vi "Go.vi"(6 "assembly type":string, 8 "First?":bool, 9 "Timing Data":T1(array[cluster]), 10 "Control In":T2={"I-O.lvclass"=refnum, "Gantry"=refnum, "Dispenser"="COM1"}, 11 "Dispense in":refnum<class "Dispense.lvclass">) -> (2 "Control Out":T2={"I-O.lvclass"=refnum, "Gantry"=refnum, "Dispenser"="COM1"}, 3 "Dispense Out":refnum<class "Dispense.lvclass">)   [LabVIEW 2021, in "Dispense.lvclass"]
uses:
  Dispense.lvclass
  Controller/Controllers.ctl
  Controller/I-O/I-O.lvclass
  C:/Program Files (x86)/Aerotech/A3200/LabVIEW/2010/Bin/Aerotech.A3200.dll
  Program Files (x86)/Aerotech/A3200/LabVIEW/2010/Bin/Aerotech.A3200.dll
  Controller/Controller.lvclass
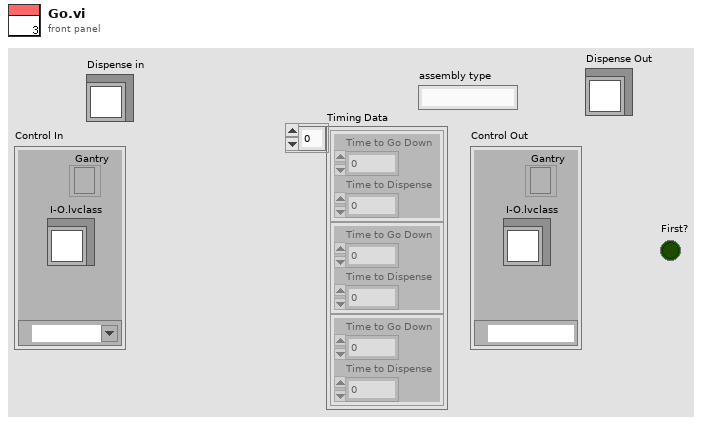
[diagram p1: front panel]
types:
  T1 = cluster{"Time to Go Down":i32, "Time to Dispense":i32}[]
  T2 = typedef "Controller.lvclass/Controllers.ctl" = cluster{"I-O.lvclass":refnum<class "I-O.lvclass">, "Gantry":refnum<k24>, "Dispenser":refnum<visa-resource-name>}
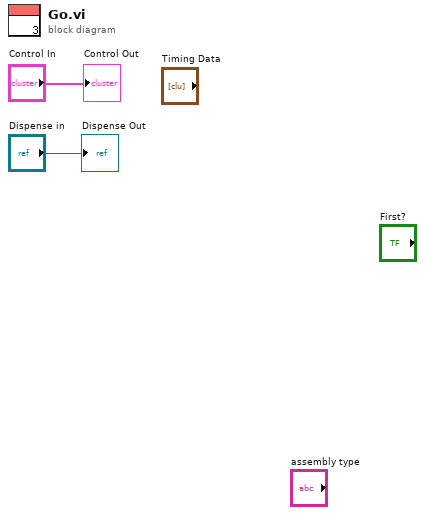
[diagram p0: block diagram]
diagram:
  "Control Out" <- "Control In"
  "Dispense Out" <- "Dispense in"
